vi "ex7-4.vi"() -> ()   [LabVIEW 2013]
panel:
  in  "x(degree)":dbl
  out "sin(x)":dbl
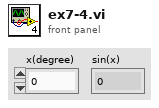
[diagram p1: front panel]
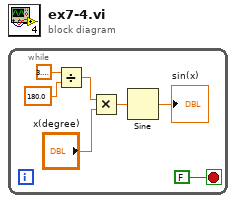
[diagram p0: block diagram]
diagram:
  n1 = while {
    stop <- FALSE stop-if-true
    n2 = Divide(x=3.141592653589793, y=180.0) -> (x/y=w5:dbl)
    n3 = Multiply(x=w5, y="x(degree)") -> (x*y=w6:dbl)
    n4 = Sine(x=w6) -> (sin(x)=→"sin(x)":dbl)
  }
